vi "VeriStand DSF.Plugin.Configuration.Create.vi"(8 "error in (no error)":errorcluster, 11 "Section Ref":T1=18446744073709551615 format="%.0x") -> (0 "error out":errorcluster, 3 "Plugin Configuration":refnum<class "VeriStand DSF.Plugin.Configuration.lvclass">)   [LabVIEW 2017, in "Data Sharing Framework Engine.lvlib" / "VeriStand DSF.Plugin.Configuration.lvclass"]
uses:
  VeriStand DSF.Plugin.Configuration.lvclass
  <vilib>/NI Veristand/Custom Device API/Custom Device API.lvlib
  DSF Core/Built/Windows/Engine/DSF.Engine.lvlibp/Shared/Classes/Plugin/DSF.Shared.Configuration.Plugin.lvclass
  VeriStand DSF.Transfer Group.Configuration.lvclass
  C:/Git/DSF/DSF Core/Built/Windows/Engine/DSF.Engine.lvlibp/Shared/Classes/Transfer Group/DSF.Shared.Configuration.Transfer Group.lvclass
  C:/Git/DSF/DSF Core/Built/Windows/Engine/DSF.Engine.lvlibp/Shared/Classes/Configuration/DSF.Shared.Configuration.lvclass
  C:/Git/DSF/DSF Core/Built/Windows/Engine/DSF.Engine.lvlibp/Shared/Classes/Plugin/DSF.Shared.Configuration.Plugin.lvclass
  <vilib>/NI Veristand/Custom Device API/Custom Device Item Ref.ctl
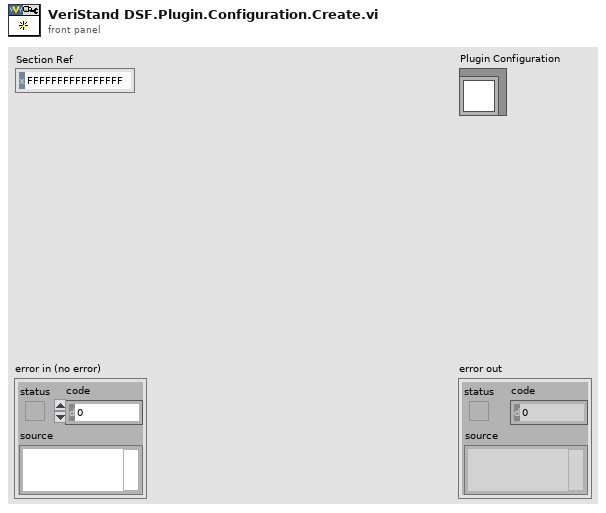
[diagram p1: front panel]
types:
  T1 = typedef "Custom Device API.lvlib/Custom Device Item Ref.ctl" = u64
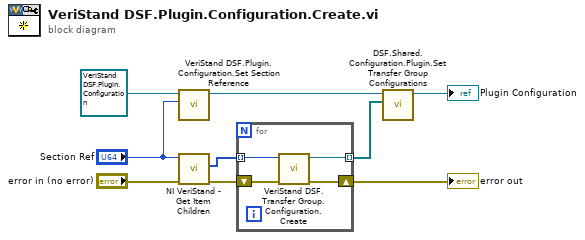
[diagram p0: block diagram]
diagram:
  n1 = call "VeriStand DSF.Plugin.Configuration.Set Section Reference.vi"("Section Ref"="Section Ref", "VeriStand DSF.Plugin.Configuration in"=refnum<class "VeriStand DSF.Plugin.Configuration.lvclass"> refnum) -> ("VeriStand DSF.Plugin.Configuration out"=w8:refnum<class "VeriStand DSF.Plugin.Configuration.lvclass">)  [unwired: 9 in]
  n2 = call <vilib>:"NI VeriStand - Get Item Children.vi"("error in (no error)"="error in (no error)", "Item Ref in"="Section Ref") -> ("error out"=w4:errorcluster, "Child Refs"=w3:T1[])  [unwired: 6 in, 2 out]
  n3 = for {
    shift-right: [w12] -> w1
    shift-left: w4 -> [w13]
    tunnel: w3 -> [w10] mode=indexing
    tunnel: [w11] -> w2 mode=indexing
    n4 = call "VeriStand DSF.Transfer Group.Configuration.Create.vi"("error in (no error)"=w13, "Section Ref"=w10) -> ("error out"=w12:errorcluster, "Transfer Group Configuration"=w11:refnum<class "VeriStand DSF.Transfer Group.Configuration.lvclass">)  [unwired: 8 in]
  }
  "error out" <- w1
  n5 = call "DSF.Shared.Configuration.Plugin.Set Transfer Group Configurations.vi"("Transfer Group Configurations"=w2, "Plugin Configuration in"=w8) -> ("Plugin Configuration out"=→"Plugin Configuration":refnum<class "VeriStand DSF.Plugin.Configuration.lvclass">)  [unwired: 9 in]
